vi "Configure Clock.vi"(8 "error in":errorcluster, 10 "Clock Source":T4(ring), 11 "Cluster":T1={"FPGA"={"Target"=enum."4", "Channel"=enum."4", "Ref1"=refnum, "Ref2"=refnum}, "10MHzRef"=FALSE, "FamInit"=0}) -> (0 "error out":errorcluster, 2 "Configuration Error":bool)   [LabVIEW 2018]
doc: "This VI configures the clock source for the NI 5762. For execution steps, refer to the comments on the block diagram."
uses:
  Controls/HWCluster.ctl
  Controls/Clusts/FPGA_Config_Clust.ctl
  Controls/Enums/TargetNumber.ctl
  <vilib>/Utility/error.llb/Error Cluster From Error Code.vi
  <vilib>/rvi/errors/niLvFpgaAdjustHostInterfaceError.vi
  <vilib>/rvi/interface/nirviReadWriteControl/nirviReadWriteControl.xnode
  <vilib>/rvi/interface/Simulation/niFpgaSimulationCallBeginRW.vi
  NiFpgaLv.dll
panel:
  # "This VI configures the clock source for the NI 5762. For execution steps, refer to the comments on the block diagram."
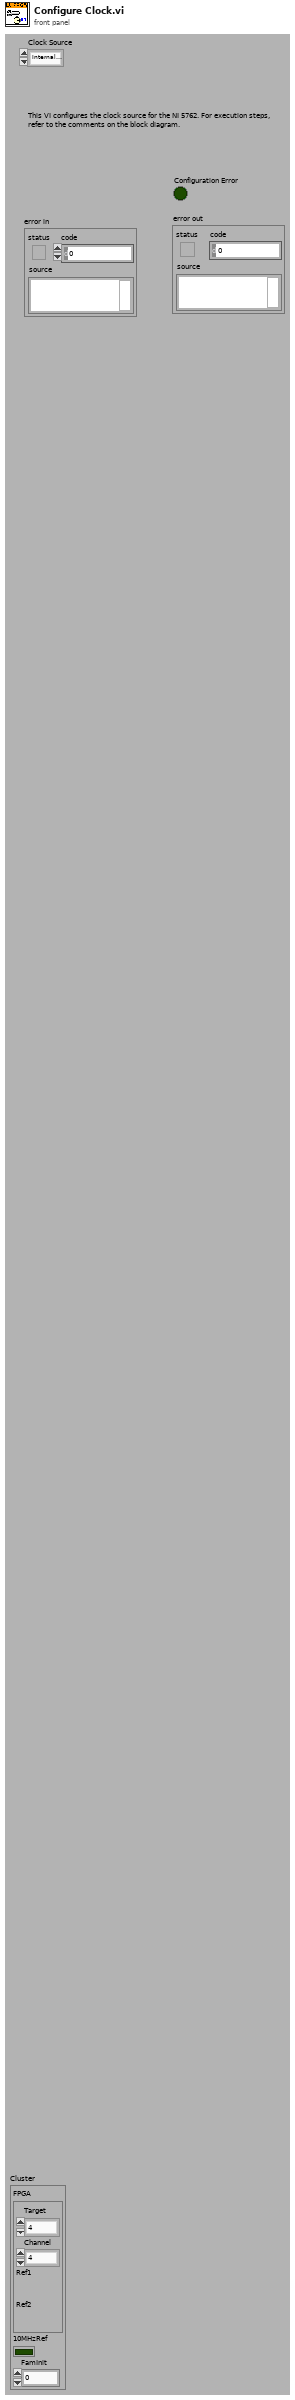
[diagram p1: front panel]
types:
  T1 = typedef "HWCluster.ctl" = cluster{"FPGA":T2, "10MHzRef":bool, "FamInit":i32}
  T2 = typedef "FPGA_Config_Clust.ctl" = cluster{"Target":T3, "Channel":T3, "Ref1":refnum<k20>, "Ref2":refnum<k20>}
  T3 = typedef "TargetNumber.ctl" = enum16{"1", "2", "3", "4"}
  T4 = enum8{"Internal Clock PLL Off", "Internal Clock PLL On (CLK_IN)", "External Clock (CLK_IN)", "Internal Clock PLL On (IoModSyncClk)"}
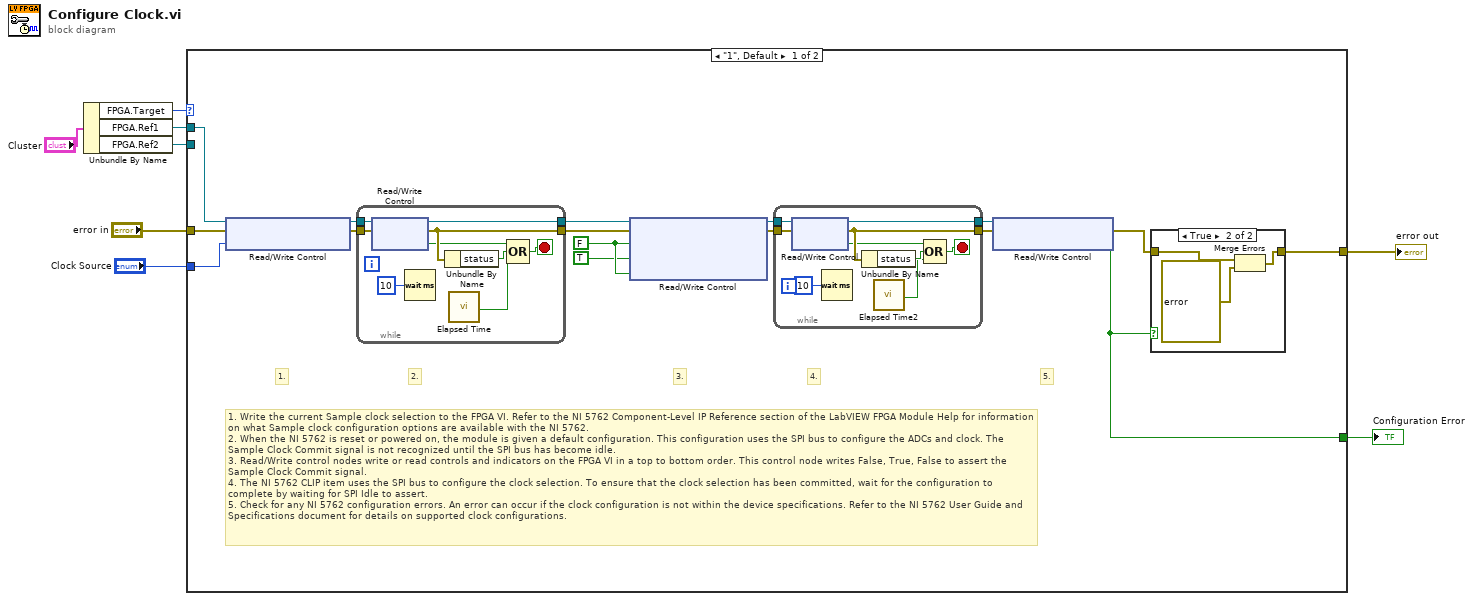
[diagram p0: block diagram]
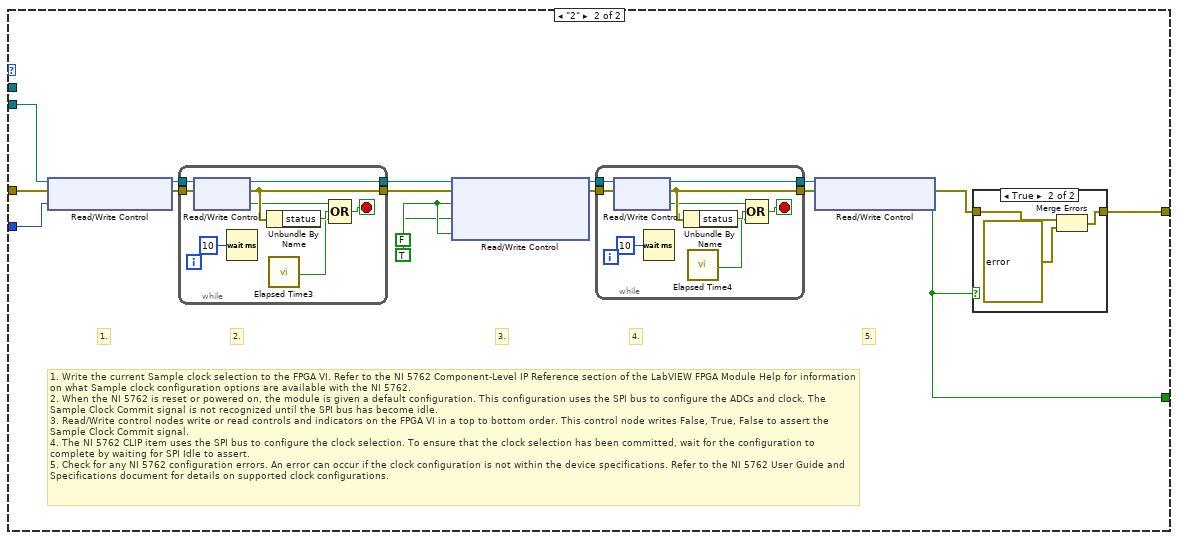
[diagram p3: hidden frame]
diagram:
  n1 = Unbundle By Name("Cluster") -> ("FPGA.Target"=w4:T3, "FPGA.Ref1"=w5:refnum<k20>, "FPGA.Ref2"=w2:refnum<k20>)
  n2 = case shown="\"1\", Default" w4 {
    tunnel: "error in" -> [w24 w62]
    tunnel: [w12 w61] -> w7
    tunnel: w5 -> [w9 _]
    tunnel: "Clock Source" -> [w11 w60]
    tunnel: w2 -> [_ w59]
    tunnel: [w10 w58] -> w1
    frame "1", Default {
      w17 = FALSE ("Sample Clock Commit")
      # "1. Write the current Sample clock selection to the FPGA VI. Refer to the NI 5762 Component-Level IP Reference section of the LabVIEW FPGA Module Help for information on what Sample clock configuration options are available with the NI 5762.\n2. When the NI 5762 is reset or powered on, the module is given a default configuration. This configuration uses the SPI bus to configure the ADCs and clock. The Sample Clock Commit signal is not recognized until the SPI bus has become idle.\n3. Read/Write control nodes write or read controls and indicators on the FPGA VI in a top to bottom order. This control node writes False, True, False to assert the Sample Clock Commit signal.\n4. The NI 5762 CLIP item uses the SPI bus to configure the clock selection. To ensure that the clock selection has been committed, wait for the configuration to complete by waiting for SPI Idle to assert.\n5. Check for any NI 5762 configuration errors. An error can occur if the clock configuration is not within the device specifications. Refer to the NI 5762 User Guide and Specifications document for details on supported clock configurations."
      # "5."
      # "4."
      # "3."
      # "2."
      # "1."
      n3 = xnode "Read/Write Control"("FPGA VI Reference In"=w9, "error in"=w24, "Sample Clock Select"=w11) -> ("FPGA VI Reference Out"=w23:refnum<k20>, "error out"=w22:errorcluster)
      n4 = while {
        tunnel: w23 -> [w42]
        tunnel: w22 -> [w43]
        tunnel: [w40] -> w20
        tunnel: [w41] -> w21
        stop <- w44 stop-if-true
        n5 = xnode "Read/Write Control"("FPGA VI Reference In"=w42, "error in"=w43) -> ("FPGA VI Reference Out"=w41:refnum<k20>, "error out"=w40:errorcluster, "SPI Idle"=w39:bool)
        n6 = Wait (ms)(milliseconds to wait=u32 10) -> ()  [unwired: 1 out]
        n7 = Unbundle By Name(w40) -> ("status"=w45:bool)
        n8 = call "Elapsed Time"() -> ("Time has Elapsed"=w38:bool)  [unwired: 12 in, 7 out]
        n9 = Compound Arithmetic op=OR(w39, w45, w38) -> (w44:bool)
      }
      n10 = xnode "Read/Write Control"("FPGA VI Reference In"=w21, "error in"=w20, "Sample Clock Commit"=w17, "Sample Clock Commit"=TRUE, "Sample Clock Commit"=w17) -> ("FPGA VI Reference Out"=w19:refnum<k20>, "error out"=w18:errorcluster)
      n11 = while {
        tunnel: w19 -> [w34]
        tunnel: w18 -> [w33]
        tunnel: [w31] -> w14
        tunnel: [w32] -> w15
        stop <- w35 stop-if-true
        n12 = xnode "Read/Write Control"("FPGA VI Reference In"=w34, "error in"=w33) -> ("FPGA VI Reference Out"=w32:refnum<k20>, "error out"=w31:errorcluster, "SPI Idle"=w30:bool)
        n13 = Wait (ms)(milliseconds to wait=u32 10) -> ()  [unwired: 1 out]
        n14 = Unbundle By Name(w31) -> ("status"=w36:bool)
        n15 = call "Elapsed Time2"() -> ("Time has Elapsed"=w29:bool)  [unwired: 12 in, 7 out]
        n16 = Compound Arithmetic op=OR(w30, w36, w29) -> (w35:bool)
      }
      n17 = xnode "Read/Write Control"("FPGA VI Reference In"=w15, "error in"=w14) -> ("error out"=w13:errorcluster, "Configuration Error"=w10:bool)  [unwired: 1 out]
      n18 = case shown="True" w10 {
        tunnel: [w25 w28] -> w12
        tunnel: w13 -> [w25 w26]
        frame False {
        }
        frame True {
          n19 = Merge Errors(w26, errorcluster {"status"=TRUE, "code"=-8998, "source"="IO Module clock not configured correctly. Please ensure that the desired clock meets the required specifications."} ("error in")) -> (w28:errorcluster)
        }
      }
    }
    frame "2" {
      w51 = FALSE ("Sample Clock Commit")
      # "1. Write the current Sample clock selection to the FPGA VI. Refer to the NI 5762 Component-Level IP Reference section of the LabVIEW FPGA Module Help for information on what Sample clock configuration options are available with the NI 5762.\n2. When the NI 5762 is reset or powered on, the module is given a default configuration. This configuration uses the SPI bus to configure the ADCs and clock. The Sample Clock Commit signal is not recognized until the SPI bus has become idle.\n3. Read/Write control nodes write or read controls and indicators on the FPGA VI in a top to bottom order. This control node writes False, True, False to assert the Sample Clock Commit signal.\n4. The NI 5762 CLIP item uses the SPI bus to configure the clock selection. To ensure that the clock selection has been committed, wait for the configuration to complete by waiting for SPI Idle to assert.\n5. Check for any NI 5762 configuration errors. An error can occur if the clock configuration is not within the device specifications. Refer to the NI 5762 User Guide and Specifications document for details on supported clock configurations."
      # "5."
      # "4."
      # "3."
      # "2."
      # "1."
      n20 = xnode "Read/Write Control"("FPGA VI Reference In"=w59, "error in"=w62, "Sample Clock Select"=w60) -> ("FPGA VI Reference Out"=w57:refnum<k20>, "error out"=w56:errorcluster)
      n21 = while {
        tunnel: w57 -> [w80]
        tunnel: w56 -> [w81]
        tunnel: [w78] -> w54
        tunnel: [w79] -> w55
        stop <- w82 stop-if-true
        n22 = xnode "Read/Write Control"("FPGA VI Reference In"=w80, "error in"=w81) -> ("FPGA VI Reference Out"=w79:refnum<k20>, "error out"=w78:errorcluster, "SPI Idle"=w77:bool)
        n23 = Wait (ms)(milliseconds to wait=u32 10) -> ()  [unwired: 1 out]
        n24 = Unbundle By Name(w78) -> ("status"=w83:bool)
        n25 = call "Elapsed Time3"() -> ("Time has Elapsed"=w76:bool)  [unwired: 12 in, 7 out]
        n26 = Compound Arithmetic op=OR(w77, w83, w76) -> (w82:bool)
      }
      n27 = xnode "Read/Write Control"("FPGA VI Reference In"=w55, "error in"=w54, "Sample Clock Commit"=w51, "Sample Clock Commit"=TRUE, "Sample Clock Commit"=w51) -> ("FPGA VI Reference Out"=w53:refnum<k20>, "error out"=w52:errorcluster)
      n28 = while {
        tunnel: w53 -> [w72]
        tunnel: w52 -> [w71]
        tunnel: [w69] -> w48
        tunnel: [w70] -> w49
        stop <- w73 stop-if-true
        n29 = xnode "Read/Write Control"("FPGA VI Reference In"=w72, "error in"=w71) -> ("FPGA VI Reference Out"=w70:refnum<k20>, "error out"=w69:errorcluster, "SPI Idle"=w68:bool)
        n30 = Wait (ms)(milliseconds to wait=u32 10) -> ()  [unwired: 1 out]
        n31 = Unbundle By Name(w69) -> ("status"=w74:bool)
        n32 = call "Elapsed Time4"() -> ("Time has Elapsed"=w67:bool)  [unwired: 12 in, 7 out]
        n33 = Compound Arithmetic op=OR(w68, w74, w67) -> (w73:bool)
      }
      n34 = xnode "Read/Write Control"("FPGA VI Reference In"=w49, "error in"=w48) -> ("error out"=w47:errorcluster, "Configuration Error"=w58:bool)  [unwired: 1 out]
      n35 = case shown="True" w58 {
        tunnel: [w63 w66] -> w61
        tunnel: w47 -> [w63 w64]
        frame False {
        }
        frame True {
          n36 = Merge Errors(w64, errorcluster {"status"=TRUE, "code"=-8998, "source"="IO Module clock not configured correctly. Please ensure that the desired clock meets the required specifications."} ("error in")) -> (w66:errorcluster)
        }
      }
    }
  }
  "error out" <- w7
  "Configuration Error" <- w1
